vi "TimeStampToString.vi"(8 "error in (no error)":errorcluster, 10 "Time Stamp":timestamp) -> (0 "error out":errorcluster, 2 "String":string)   [LabVIEW 2015, in "Request.lvclass"]
uses:
  Request.lvclass
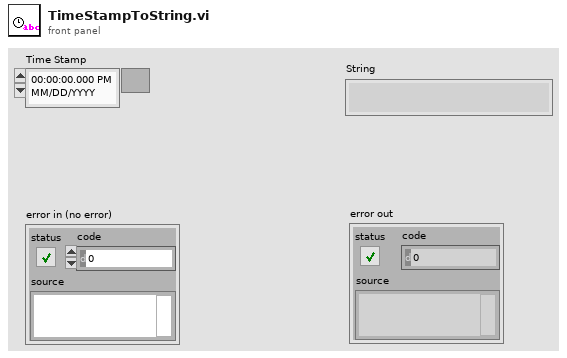
[diagram p1: front panel]
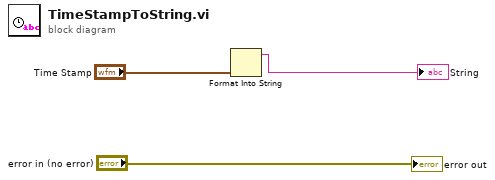
[diagram p0: block diagram]
diagram:
  n1 = Format Into String("Time Stamp") -> (resulting string=→"String":string)  [unwired: 3 in, 1 out]
  "error out" <- "error in (no error)"
